vi "Execution Start.vi"(8 "error in (no error)":errorcluster, 10 "Execution in":refnum<data-value>, 11 "Plugin in":refnum<class "Plugin.lvclass">) -> (0 "error out":errorcluster, 2 "Execution out":refnum<data-value>, 3 "Plugin out":refnum<class "Plugin.lvclass">)   [LabVIEW 2015, in "Plugin.lvclass"]
uses:
  Plugin.lvclass
  Execution.lvclass
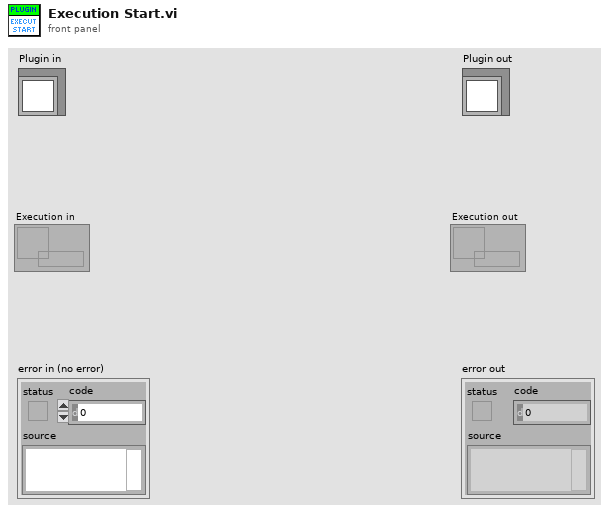
[diagram p1: front panel]
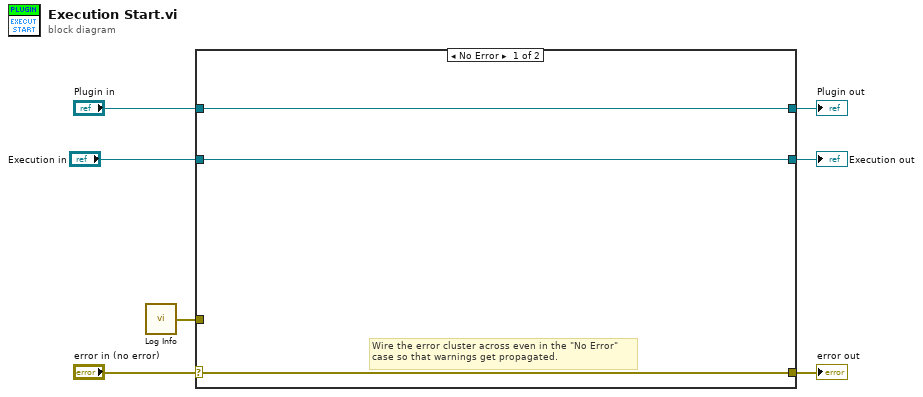
[diagram p0: block diagram]
diagram:
  n1 = call "Log Info.vi"() -> ("error out"=w1:errorcluster)  [unwired: 5 in]
  n2 = case shown="No Error" "error in (no error)" {
    selector: "error in (no error)" -> [w9 w13]
    tunnel: [w9 w13] -> w6
    tunnel: [w10 w12] -> w4
    tunnel: "Plugin in" -> [w10 w12]
    tunnel: "Execution in" -> [w8 w11]
    tunnel: [w8 w11] -> w2
    tunnel: w1 -> [_ _]
    frame No Error {
      # "Wire the error cluster across even in the \"No Error\"\ncase so that warnings get propagated."
    }
    frame Error {
    }
  }
  "error out" <- w6
  "Plugin out" <- w4
  "Execution out" <- w2
